vi "Cache-StatusChangeEventRef.vi"(8 "error in (no error)":errorcluster, 11 "Name (\"\" to Use UUID) In":string) -> (0 "error out":errorcluster, 2 "Interrupt Event":refnum<user-event>, 3 "Status Event":refnum<user-event>)   [LabVIEW 2017, in "Communicable State Machine.lvlib"]
uses:
  Communicable State Machine.lvlib
  Typedef/_CSM Status Change Event Data.ctl
  CSMQ/_CSMOFGVOPER.ctl
  ChangeFlag/ChangeFlag-Read.vi
  ChangeFlag/ChangeFlagDB.vi
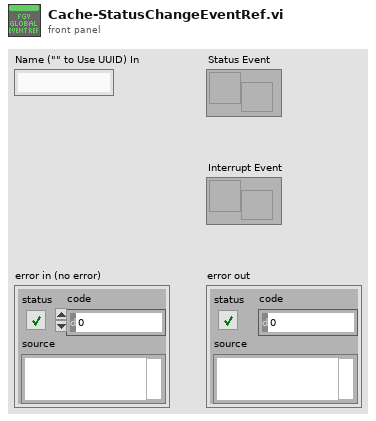
[diagram p1: front panel]
types:
  T1 = typedef "Communicable State Machine.lvlib/_CSMOFGVOPER.ctl" = enum16{"Create If not Exist", "Get By Name", "List", "Check If Name Exists", "Release", "Module Status", "Create Status Event Handler", "Destroy Status Event Handler", "Clear Invalid Objs"}
  T2 = typedef "Communicable State Machine.lvlib/_CSMObj.ctl" = cluster{"info":T3, "Refs":T5}
  T3 = typedef "Communicable State Machine.lvlib/_CSMObj-Info.ctl" = cluster{"Module Name":string, "Requested Name":string, "Group Name":string, "Mode":T4, "Allowed Messages":string[]}
  T4 = typedef "Communicable State Machine.lvlib/_CSM_MODE.ctl" = enum16{"Not Exist", "Stand Alone", "CSM", "Worker", "Worker Agent", "Chain Node", "Chain"}
  T5 = typedef "Communicable State Machine.lvlib/_CSMObj-Refs.ctl" = cluster{"WatchDogQ":refnum<queue>, "CSMDataDVR":refnum<data-value>, "Queue":T6, "GroupDataDVR":refnum<data-value>, "TagMap":refnum<data-value>, "ExitEvent":refnum<user-event>, "NewStateEvent":refnum<user-event>, "StatusEvent":refnum<user-event>, "InterruptEvent":refnum<user-event>}
  T6 = typedef "Communicable State Machine.lvlib/Priority Queue.ctl" = cluster{"HPriorityQ":refnum<queue>, "LowPriorityQ":refnum<queue>}
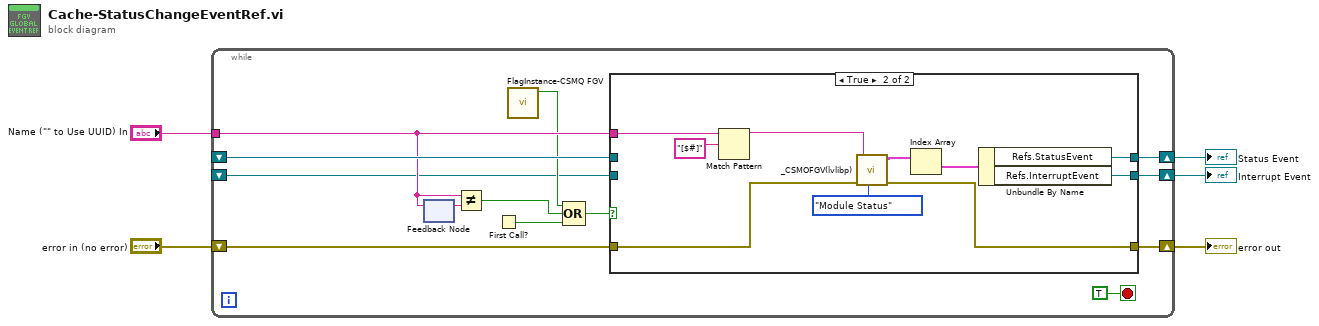
[diagram p0: block diagram]
diagram:
  n1 = while {
    shift-right: [w16] -> w3
    shift-left: "error in (no error)" -> [w17]
    shift-right: [w18] -> w5
    shift-left: _ -> [w14]
    tunnel: "Name (\"\" to Use UUID) In" -> [w13]
    shift-right: [w7] -> w1
    shift-left: _ -> [w6]
    stop <- TRUE stop-if-true
    n2 = feedback-in #1(w13) -> ()
    n3 = feedback #1() -> (w12:string)  [unwired: 1 in]
    n4 = Not Equal?(x=w13, y=w12) -> (x != y?=w11:bool)
    n5 = First Call?() -> (First Call?: T/F=w9:bool)
    n6 = call "FlagInstance-CSMQ FGV.vi"() -> ("Changed"=w8:bool)  [unwired: 10 in, 1 out]
    n7 = Compound Arithmetic op=OR(w8, w11, w9) -> (w10:bool)
    n8 = case shown="True" w10 {
      tunnel: [w21 w26] -> w18
      tunnel: w17 -> [w20 w29]
      tunnel: [w20 w30] -> w16
      tunnel: w14 -> [w21 _]
      tunnel: w13 -> [_ w25]
      tunnel: [w19 w22] -> w7
      tunnel: w6 -> [w19 _]
      frame False {
      }
      frame True {
        n9 = Match Pattern(string=w25, regular expression="[$#]") -> (before substring=w24:string)  [unwired: 1 in, 3 out]
        n10 = call "_CSMOFGV(lvlibp).vi"("Operation"=_CSMOFGVOPER."Module Status", "Error In"=w29, "Name (\"\" to Use UUID) In"=w24) -> ("error out"=w30:errorcluster, "Array"=w28:T2[])  [unwired: 6 in, 1 out]
        n11 = Index Array(array=w28) -> (element=w27:T2)  [unwired: 1 in]
        n12 = Unbundle By Name(w27) -> ("Refs.StatusEvent"=w26:refnum<user-event>, "Refs.InterruptEvent"=w22:refnum<user-event>)
      }
    }
  }
  "Status Event" <- w5
  "error out" <- w3
  "Interrupt Event" <- w1
